vi "Save Digital Data.vi"(8 "error in (no error)":errorcluster, 10 "Data Cluster":cluster{"Path":path, "Array":bool[]}, 11 "CSV in":refnum<class "CSV.lvclass">) -> (0 "error out":errorcluster, 3 "CSV out":refnum<class "CSV.lvclass">)   [LabVIEW 2020, in "CSV.lvlib" / "CSV.lvclass"]
uses:
  CSV.lvclass
  <vilib>/Utility/file.llb/Write Delimited Spreadsheet (I64).vi
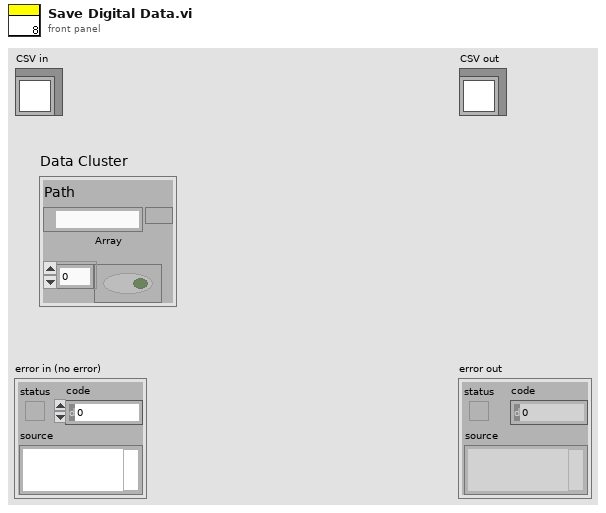
[diagram p1: front panel]
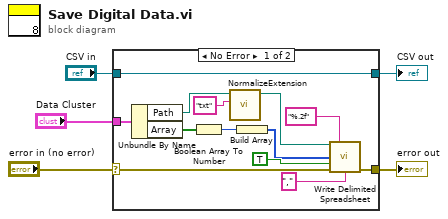
[diagram p0: block diagram]
diagram:
  n1 = case shown="No Error" "error in (no error)" {
    selector: "error in (no error)" -> [w14 w19]
    tunnel: "CSV in" -> [w18 w20]
    tunnel: [w18 w20] -> w4
    tunnel: [w15 w19] -> w3
    tunnel: "Data Cluster" -> [w10 _]
    frame No Error {
      n2 = Unbundle By Name(w10) -> ("Path"=w9:path, "Array"=w8:bool[])
      n3 = Boolean Array To Number(Boolean array=w8) -> (number=w7:u32)
      n4 = call "NormalizeExtension.vi"("Extension"="txt", "Path in"=w9) -> ("Path out"=w16:path)  [unwired: 9 in]
      n5 = Build Array(w7) -> (w6:u32[])
      n6 = call-poly <vilib>:"Write Delimited Spreadsheet.vi"("file path (dialog if empty)"=w16, "format (%d)"="%.2f" ("format (%.3f)"), "1D data"=w6, "append to file? (new file:F)"=TRUE, "error in (no error)"=w14, "delimiter (\\t)"="," ("delimiter (\\t)")) -> ("error out"=w15:errorcluster)  [unwired: 8 in, 1 out]
    }
    frame Error {
    }
  }
  "error out" <- w3
  "CSV out" <- w4
